vi "Seq Dialog Check RSLinx Tag String.vi"(8 "Segment Data":T3) -> (0 "Step Hisitory":string[](array[string]), 2 "Segment Data 2":T3)   [LabVIEW 2018]
uses:
  type defs/plc path and tag.ctl
  <vilib>/Platform/dataskt.llb/DataSocket Reference Type.ctl
  type defs/Sequence Info.ctl
  type defs/RSLinx String Cluster.ctl
panel:
  in  "timeout (ms)":i32=10000
  in  "Error No.":u16=157
  in  "Data String":string
  in  "Tag String":T1={"Tag Name"="S060.PXI.Signals.PlltData.SN", "Network Path"="172.15.51.1,1,0", "use opc"=FALSE, "DataSocket Reference"={"CWDSLib._DCWDataSocket"=refnum, "CWDSLib._DCWData"=refnum, "OnDataUpdated"=0, "OnStatusUpdated"=0}} {"DataSocket Reference"."OnStatusUpdated" format="%.0x"; "DataSocket Reference"."OnDataUpdated" format="%.0x"}
  out "Name":string="Pre Run Station - Glass - Vent Open"
  in  "Description":string
  in  "Save":bool
  in  "Cancel":bool
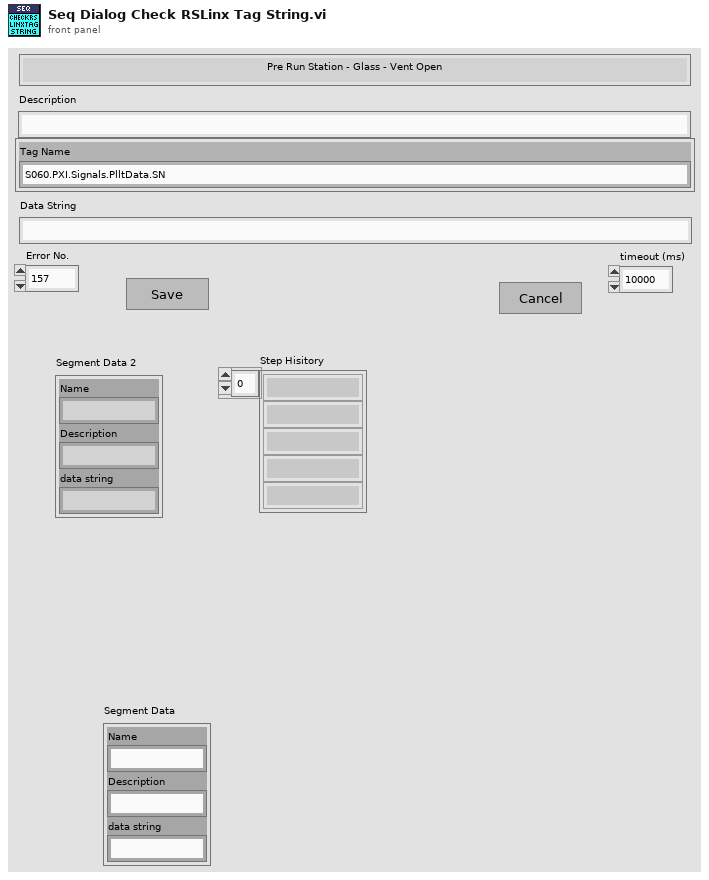
[diagram p1: front panel]
types:
  T1 = typedef "plc path and tag.ctl" = cluster{"Tag Name":string, "Network Path":string, "use opc":bool, "DataSocket Reference":T2}
  T2 = typedef "DataSocket Reference Type.ctl" = cluster{"CWDSLib._DCWDataSocket":refnum<k7>, "CWDSLib._DCWData":refnum<k7>, "OnDataUpdated":u32, "OnStatusUpdated":u32}
  T3 = typedef "Sequence Info.ctl" = cluster{"Name":string, "Description":string, "data string":string}
  T4 = typedef "RSLinx String Cluster.ctl" = cluster{"Data String":string, "PLC Path and Tag":T1, "Error No.":u16, "timeout (ms)":i32}
  T5 = cluster{"Segment Data":T3, "Old Data":string, "New Data":string, "RSLinx String Cluster":T4}
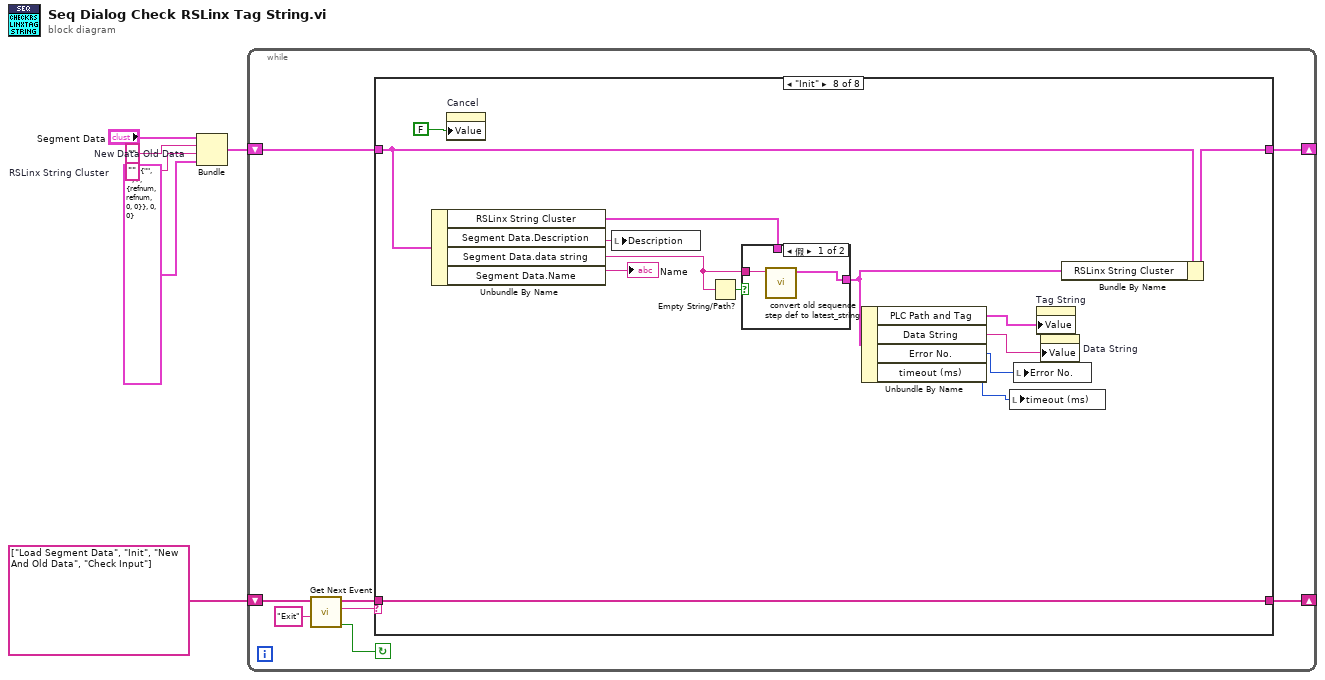
[diagram p0: block diagram]
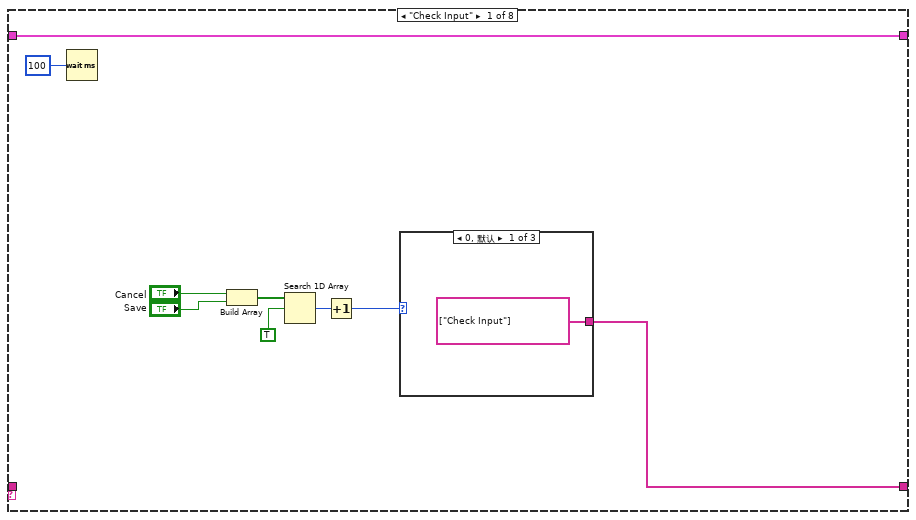
[diagram p2: hidden frame]
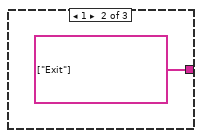
[diagram p3: hidden frame]
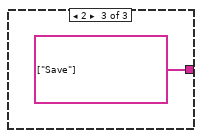
[diagram p4: hidden frame]
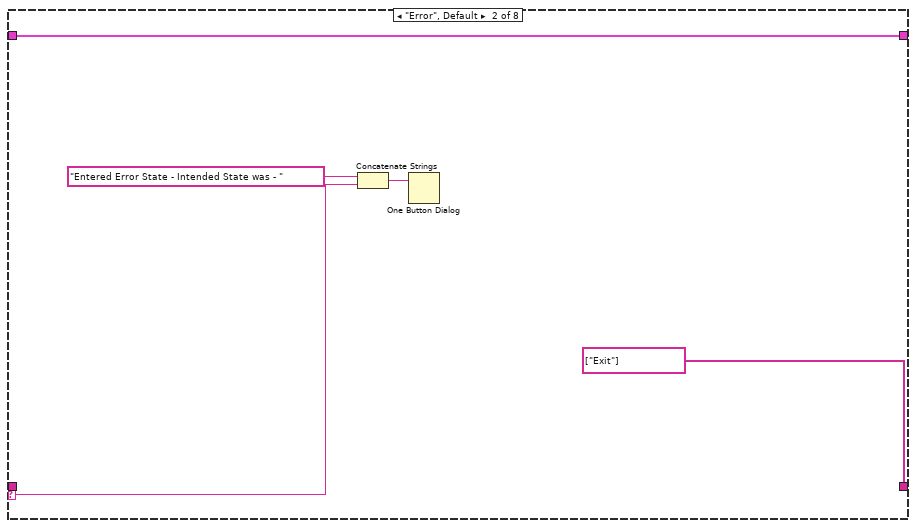
[diagram p5: hidden frame]
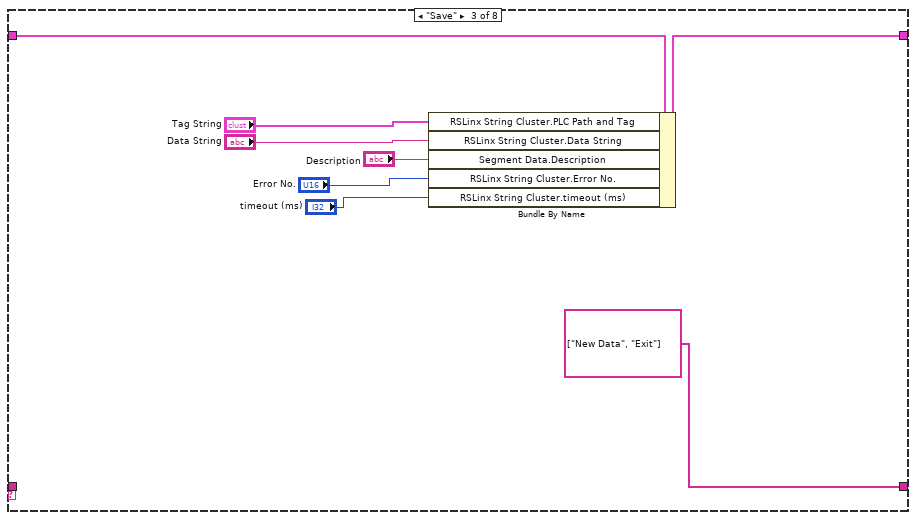
[diagram p6: hidden frame]
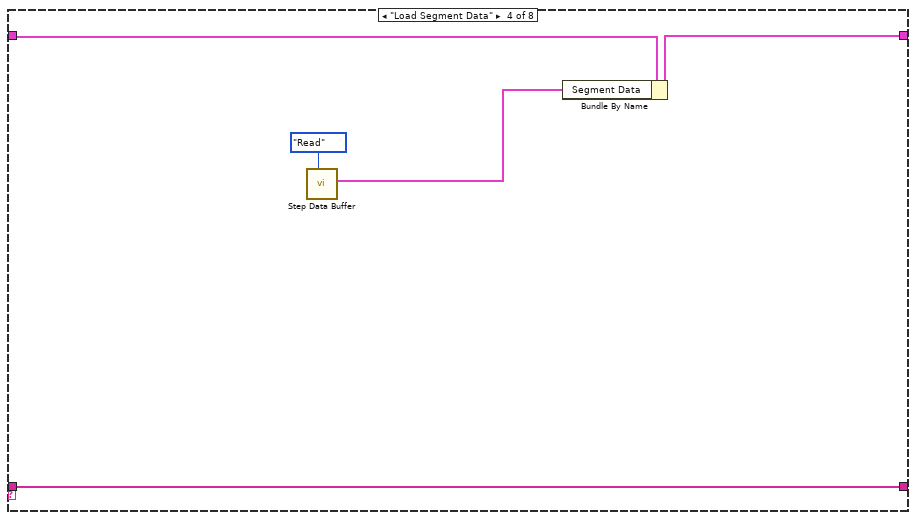
[diagram p7: hidden frame]
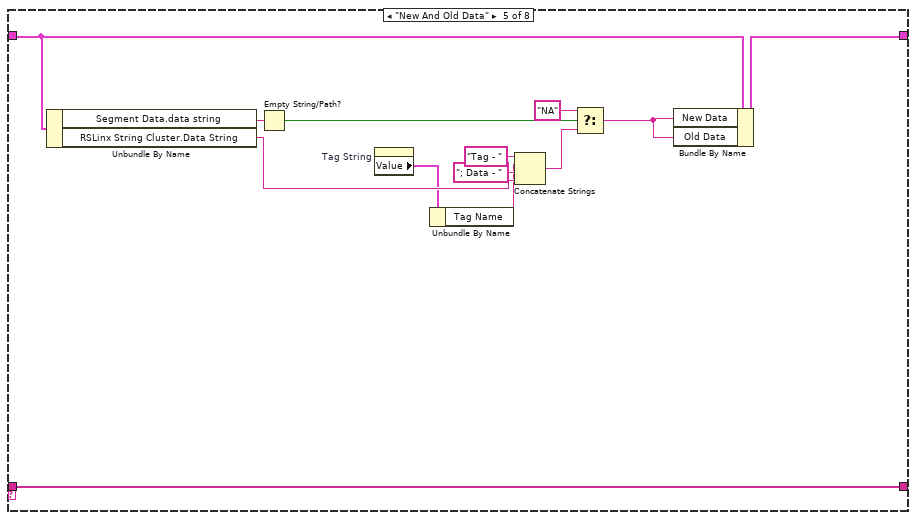
[diagram p8: hidden frame]
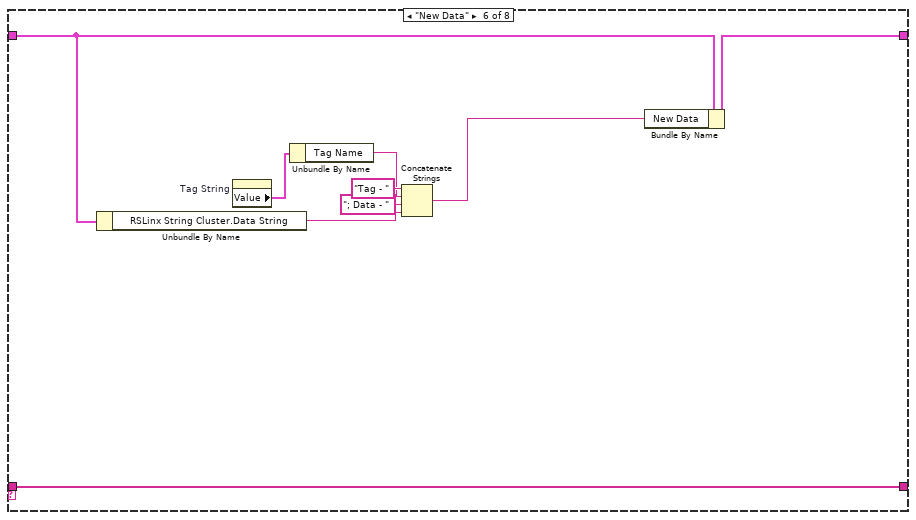
[diagram p9: hidden frame]
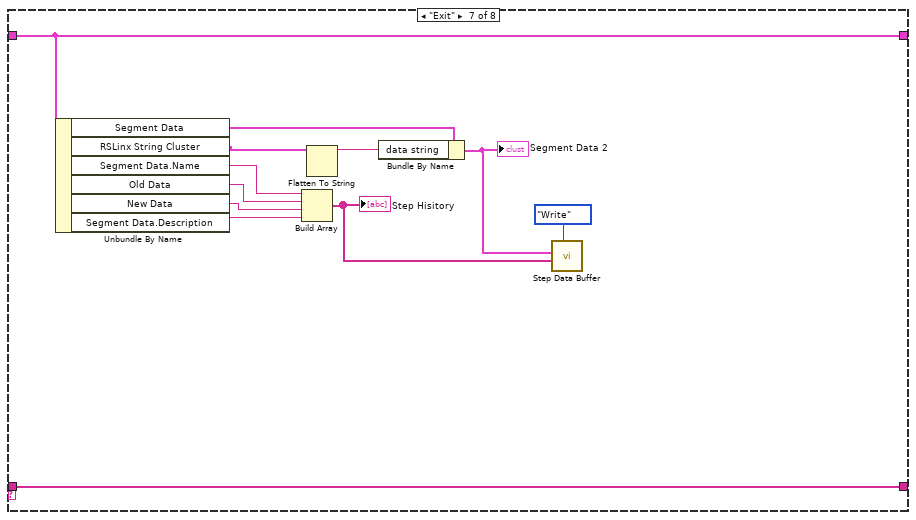
[diagram p10: hidden frame]
diagram:
  w1 = T4 {"Data String"="", "PLC Path and Tag"={"Tag Name"="", "Network Path"="", "use opc"=FALSE, "DataSocket Reference"={"CWDSLib._DCWDataSocket"=refnum, "CWDSLib._DCWData"=refnum, "OnDataUpdated"=0, "OnStatusUpdated"=0}}, "Error No."=0, "timeout (ms)"=0}  # RSLinx String Cluster
  w3 = ""  # New Data
  w4 = ""  # Old Data
  n1 = Bundle("Segment Data"="Segment Data", "Old Data"=w4, "New Data"=w3, "RSLinx String Cluster"=w1) -> (w6:T5)  [unwired: 1 in]
  n2 = while {
    shift-right: [w12] -> _
    shift-left: string[] ["Load Segment Data", "Init", "New And Old Data", "Check Input"] ("Event queue out") -> [w11]
    shift-right: [w7] -> _
    shift-left: w6 -> [w8]
    stop <- w10 continue-if-true
    n3 = call "Get Next Event.vi"("Exit Event"="Exit", "event queue in"=w11) -> ("Condition (Exit:F)"=w10:bool, "next event"=w14:string, "event queue out"=w13:string[])  [unwired: 3 in]
    n4 = case shown="\"Init\"" w14 {
      selector: w14 -> [_ w29 _ _ _ _ _ _]
      tunnel: w13 -> [_ _ _ w40 w51 w66 w78 w92]
      tunnel: [w17 string[] ["Exit"] ("event queue out") string[] ["New Data", "Exit"] ("Event queue out") w40 w51 w66 w78 w92] -> w12
      tunnel: w8 -> [w22 w27 w38 w42 w53 w65 w77 w87]
      tunnel: [w22 w27 w39 w41 w52 w64 w77 w84] -> w7
      frame "Check Input" {
        n5 = Wait (ms)(milliseconds to wait=u32 100) -> ()  [unwired: 1 out]
        n6 = Build Array("Cancel", "Save") -> (w19:bool[])
        n7 = Search 1D Array(1D array=w19, element=TRUE) -> (index of element=w20:i32)  [unwired: 1 in]
        n8 = Increment(x=w20) -> (x+1=w21:i32)
        n9 = case shown="0, 默认" w21 {
          tunnel: [string[] ["Check Input"] ("Events to Insert") string[] ["Exit"] ("Events to Insert") string[] ["Save"] ("Events to Insert")] -> w17
          frame 0, Default {
          }
          frame 1 {
          }
          frame 2 {
          }
        }
      }
      frame "Error", Default {
        n10 = Concatenate Strings("Entered Error State - Intended State was - " ("string"), w29) -> (w31:string)
        n11 = One Button Dialog(message=w31) -> ()  [unwired: 1 in, 1 out]
      }
      frame "Save" {
        n12 = Bundle By Name(cluster=w38, "RSLinx String Cluster.PLC Path and Tag"="Tag String", "RSLinx String Cluster.Data String"="Data String", "Segment Data.Description"="Description", "RSLinx String Cluster.Error No."="Error No.", "RSLinx String Cluster.timeout (ms)"="timeout (ms)") -> (w39:T5)
      }
      frame "Load Segment Data" {
        n13 = call "Step Data Buffer.vi"("Mode"=enum16{"Init", "Read", "Write"}."Read") -> ("Segment Data Out"=w44:T3)  [unwired: 6 in, 4 out]
        n14 = Bundle By Name(cluster=w42, "Segment Data"=w44) -> (w41:T5)
      }
      frame "New And Old Data" {
        n15 = Unbundle By Name(w53) -> ("Segment Data.data string"=w57:string, "RSLinx String Cluster.Data String"=w48:string)
        n16 = Empty String/Path?(string/path=w57) -> (empty?=w54:bool)
        n17 = property on="Tag String" class="Clust (严格)"() -> ("Value"=w46:T1)  [unwired: 2 in, 2 out]
        n18 = Unbundle By Name(w46) -> ("Tag Name"=w45:string)
        n19 = Concatenate Strings("Tag - " ("string"), w45, "; Data - " ("string"), w48) -> (w47:string)
        n20 = Select(t="NA", s=w54, f=w47) -> (s? t:f=w56:string)
        n21 = Bundle By Name(cluster=w53, "New Data"=w56, "Old Data"=w56) -> (w52:T5)
      }
      frame "New Data" {
        n22 = Unbundle By Name(w65) -> ("RSLinx String Cluster.Data String"=w61:string)
        n23 = property on="Tag String" class="Clust (严格)"() -> ("Value"=w59:T1)  [unwired: 2 in, 2 out]
        n24 = Unbundle By Name(w59) -> ("Tag Name"=w58:string)
        n25 = Concatenate Strings("Tag - " ("string"), w58, "; Data - " ("string"), w61) -> (w60:string)
        n26 = Bundle By Name(cluster=w65, "New Data"=w60) -> (w64:T5)
      }
      frame "Exit" {
        n27 = Unbundle By Name(w77) -> ("Segment Data"=w67:T3, "RSLinx String Cluster"=w68:T4, "Segment Data.Name"=w76:string, "Old Data"=w75:string, "New Data"=w74:string, "Segment Data.Description"=w71:string)
        n28 = Build Array(w76, w75, w74, w71) -> (w72:string[])
        "Step Hisitory" <- w72
        n29 = Flatten To String(anything=w68) -> (data string=w70:string)  [unwired: 3 in, 2 out]
        n30 = Bundle By Name(cluster=w67, "data string"=w70) -> (w69:T3)
        "Segment Data 2" <- w69
        n31 = call "Step Data Buffer.vi"("Mode"=enum16{"Init", "Read", "Write"}."Write", "Step Hisitory In"=w72, "Segment Data In"=w69) -> ()  [unwired: 4 in, 5 out]
      }
      frame "Init" {
        n32 = Unbundle By Name(w87) -> ("RSLinx String Cluster"=w88:T4, "Segment Data.Description"=w91:string, "Segment Data.data string"=w85:string, "Segment Data.Name"=→"Name":string)
        n33 = property on="Cancel" class="Bool (严格)"("Value"=FALSE ("Cancel")) -> ()  [unwired: 2 in, 2 out]
        n34 = local write "Description"(w91) -> ()
        n35 = Empty String/Path?(string/path=w85) -> (empty?=w86:bool)
        n36 = case shown="假" w86 {
          tunnel: w85 -> [w93 _]
          tunnel: w88 -> [_ w95]
          tunnel: [w94 w95] -> w81
          frame False {
            n37 = call "convert old sequence step def to latest_string.vi"("data string"=w93) -> ("RSLinx String Cluster out"=w94:T4)  [unwired: 9 in, 1 out]
          }
          frame True {
          }
        }
        n38 = Unbundle By Name(w81) -> ("PLC Path and Tag"=w83:T1, "Data String"=w82:string, "Error No."=w80:u16, "timeout (ms)"=w79:i32)
        n39 = local write "timeout (ms)"(w79) -> ()
        n40 = local write "Error No."(w80) -> ()
        n41 = property on="Tag String" class="Clust (严格)"("Value"=w83) -> ()  [unwired: 2 in, 2 out]
        n42 = property on="Data String" class="Str"("Value"=w82) -> ()  [unwired: 2 in, 2 out]
        n43 = Bundle By Name(cluster=w87, "RSLinx String Cluster"=w81) -> (w84:T5)
      }
    }
  }
